vi "Check on event_REMAKE.vi"(7 "Derivative Threshold":dbl=0.02 min=0.0 max=0.5 step=0.01 format="%#_6gV", 8 "Error In":errorcluster, 9 "YPR data":sgl[](array[numeric])=[0.0, 0.0, 0.0, 0.0, 0.0, 0.0, 0.0, 0.0, 0.0, 0.0, 0.0, 0.0], 10 "Strain data":sgl[](array[numeric])=[0.0, 0.0, 0.0, 0.0, 0.0, 0.0, 0.0, 0.0, 0.0, 0.0, 0.0, 0.0], 11 "Event cluster in":T1) -> (0 "Error Out":errorcluster, 1 "event ongoing":bool, 2 "new event finished":bool, 3 "Event cluster":T1)   [LabVIEW 2016]
uses:
  Typedef/Event cluster.ctl
  Typedef/SVM train class.ctl
  Typedef/SVM predict class.ctl
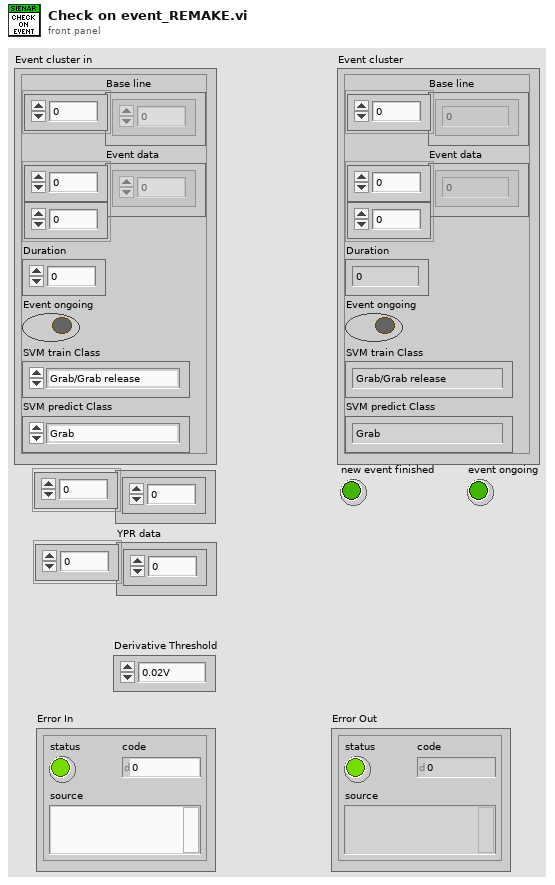
[diagram p1: front panel]
types:
  T1 = typedef "Event cluster.ctl" = cluster{"Base line":dbl[], "Event data":dbl[][], "Duration":dbl, "Event ongoing":bool, "SVM train Class":T2, "SVM predict Class":T3}
  T2 = typedef "SVM train class.ctl" = enum16{"Grab/Grab release", "Hand flexion/HF release", "Hand extension/HE release", "Tap", "Swipe_CW", "Swipe_CCW"}
  T3 = typedef "SVM predict class.ctl" = enum16{"Grab", "Grab release", "Hand flexion", "Hand flexion release", "Hand extension", "Hand extension release", "Tap", "Swipe_CW", "Swipe_CCW"}
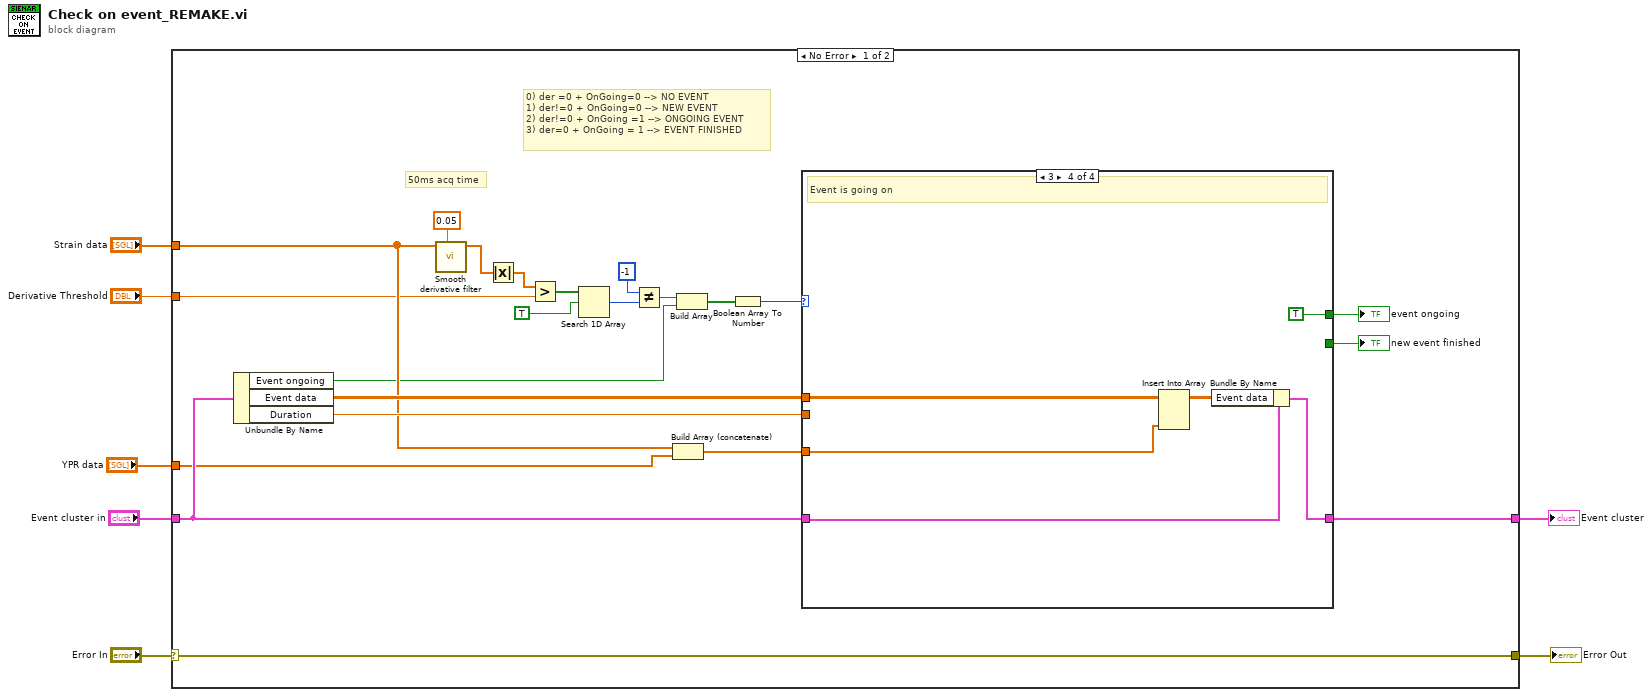
[diagram p0: block diagram]
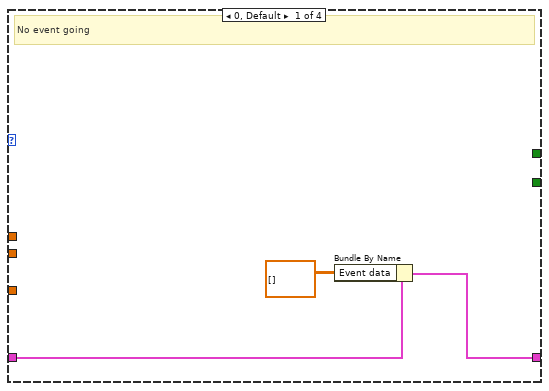
[diagram p2: hidden frame]
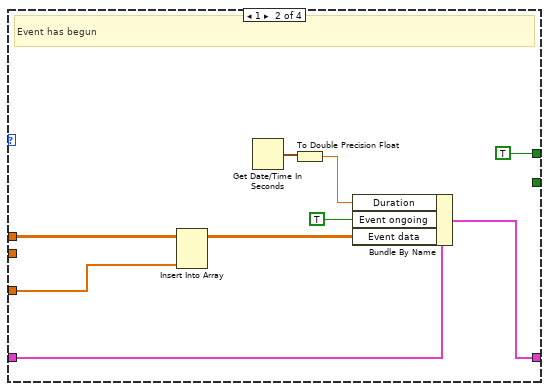
[diagram p3: hidden frame]
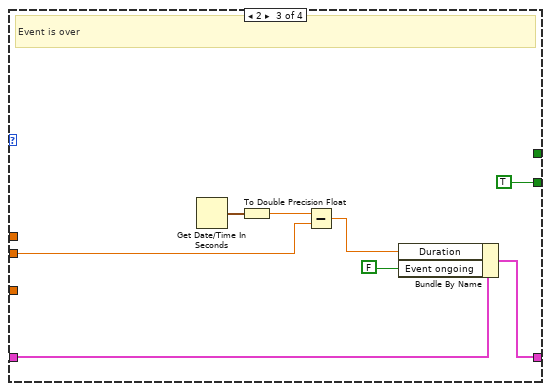
[diagram p4: hidden frame]
diagram:
  n1 = case shown="No Error" "Error In" {
    selector: "Error In" -> [w26 w56]
    tunnel: "Event cluster in" -> [w29 w57]
    tunnel: "Derivative Threshold" -> [w19 _]
    tunnel: "Strain data" -> [w20 _]
    tunnel: [w28 w57] -> w2
    tunnel: [w26 w56] -> w3
    tunnel: "YPR data" -> [w23 _]
    frame No Error {
      # "0) der =0 + OnGoing=0 --> NO EVENT\n1) der!=0 + OnGoing=0 --> NEW EVENT\n2) der!=0 + OnGoing =1 --> ONGOING EVENT\n3) der=0 + OnGoing = 1 --> EVENT FINISHED"
      # "50ms acq time"
      n2 = Unbundle By Name(w29) -> ("Event ongoing"=w16:bool, "Event data"=w27:dbl[][], "Duration"=w25:dbl)
      n3 = call "Smooth derivative filter.vi"("dt"=0.05, "Strain data"=w20) -> ("dStrain/dt"=w17:dbl[])  [unwired: 8 in, 1 out]
      n4 = Absolute Value(x=w17) -> (abs(x)=w8:dbl[])
      n5 = Greater?(x=w8, y=w19) -> (0:w15:bool[])
      n6 = Search 1D Array(1D array=w15, element=TRUE) -> (index of element=w13:i32)  [unwired: 1 in]
      n7 = Not Equal?(x=-1, y=w13) -> (x != y?=w11:bool)
      n8 = Build Array (concatenate)(w20, w23) -> (w22:sgl[])
      n9 = Build Array(w11, w16) -> (w10:bool[])
      n10 = Boolean Array To Number(Boolean array=w10) -> (number=w9:u32)
      n11 = case shown="3" w9 {
        tunnel: w29 -> [w32 w41 w48 w53]
        tunnel: [w31 w40 w47 w54] -> w28
        tunnel: w27 -> [_ w38 _ w55]
        tunnel: w25 -> [_ _ w44 _]
        tunnel: [_ _ TRUE _] -> w24
        tunnel: w22 -> [_ w34 _ w51]
        tunnel: [_ TRUE _ TRUE] -> w21
        frame 0, Default {
          # "No event going"
          n12 = Bundle By Name(cluster=w32, "Event data"=dbl[][] []) -> (w31:T1)
        }
        frame 1 {
          # "Event has begun"
          n13 = Insert Into Array(array=w38, new element=w34) -> (w37:dbl[][])  [unwired: 2 in]
          n14 = Get Date/Time In Seconds() -> (seconds since 1Jan1904=w36:timestamp)
          n15 = To Double Precision Float(number=w36) -> (double precision float=w35:dbl)
          n16 = Bundle By Name(cluster=w41, "Duration"=w35, "Event ongoing"=TRUE, "Event data"=w37) -> (w40:T1)
        }
        frame 2 {
          # "Event is over"
          n17 = Get Date/Time In Seconds() -> (seconds since 1Jan1904=w46:timestamp)
          n18 = To Double Precision Float(number=w46) -> (double precision float=w45:dbl)
          n19 = Subtract(x=w45, y=w44) -> (x-y=w43:dbl)
          n20 = Bundle By Name(cluster=w48, "Duration"=w43, "Event ongoing"=FALSE) -> (w47:T1)
        }
        frame 3 {
          # "Event is going on"
          n21 = Insert Into Array(array=w55, new element=w51) -> (w52:dbl[][])  [unwired: 2 in]
          n22 = Bundle By Name(cluster=w53, "Event data"=w52) -> (w54:T1)
        }
      }
      "new event finished" <- w24
      "event ongoing" <- w21
    }
    frame Error {
    }
  }
  "Error Out" <- w3
  "Event cluster" <- w2
